vi "Calibrate Ticks 2 Timeouts (uSMC).vi"(0 "Buttons Timeout 1 (ticks)":u16=4262, 1 "Reduce Current Timeout (ticks)":u16=6458, 5 "Buttons Timeout 2 (ticks)":u16=12916, 7 "Buttons Timeout 3 (ticks)":u16=12916, 9 "Buttons Timeout 4 (ticks)":u16=12916, 11 "Buttons Timeout Reset (ticks)":u16=9687, 12 "Buttons Timeout DblClick (ticks)":u16=1937) -> (3 "Reduce Current Timeout (ms)":u16, 4 "Buttons Timeout 1 (ms)":u16, 6 "Buttons Timeout 2 (ms)":u16, 8 "Buttons Timeout 3 (ms)":u16, 10 "Buttons Timeout 4 (ms)":u16, 14 "Buttons Timeout DblClick (ms)":u16, 15 "Buttons Timeout Reset (ms)":u16)   [LabVIEW 2010, in "SignalWriterMH110203USBStepperMotor.lvclass"]
uses:
  SignalWriterMH110203USBStepperMotor.lvclass
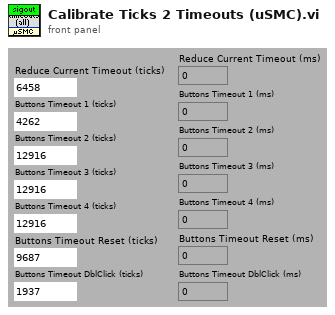
[diagram p1: front panel]
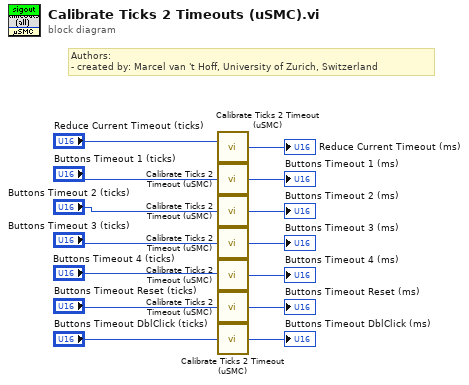
[diagram p0: block diagram]
diagram:
  # "Authors: \n- created by: Marcel van 't Hoff, University of Zurich, Switzerland"
  n1 = call "Calibrate Ticks 2 Timeout (uSMC).vi"("Timeouts (Ticks)"="Reduce Current Timeout (ticks)") -> ("Timeout (ms)"=→"Reduce Current Timeout (ms)":u16)
  n2 = call "Calibrate Ticks 2 Timeout (uSMC).vi"("Timeouts (Ticks)"="Buttons Timeout 1 (ticks)") -> ("Timeout (ms)"=→"Buttons Timeout 1 (ms)":u16)
  n3 = call "Calibrate Ticks 2 Timeout (uSMC).vi"("Timeouts (Ticks)"="Buttons Timeout 2 (ticks)") -> ("Timeout (ms)"=→"Buttons Timeout 2 (ms)":u16)
  n4 = call "Calibrate Ticks 2 Timeout (uSMC).vi"("Timeouts (Ticks)"="Buttons Timeout 3 (ticks)") -> ("Timeout (ms)"=→"Buttons Timeout 3 (ms)":u16)
  n5 = call "Calibrate Ticks 2 Timeout (uSMC).vi"("Timeouts (Ticks)"="Buttons Timeout 4 (ticks)") -> ("Timeout (ms)"=→"Buttons Timeout 4 (ms)":u16)
  n6 = call "Calibrate Ticks 2 Timeout (uSMC).vi"("Timeouts (Ticks)"="Buttons Timeout Reset (ticks)") -> ("Timeout (ms)"=→"Buttons Timeout Reset (ms)":u16)
  n7 = call "Calibrate Ticks 2 Timeout (uSMC).vi"("Timeouts (Ticks)"="Buttons Timeout DblClick (ticks)") -> ("Timeout (ms)"=→"Buttons Timeout DblClick (ms)":u16)
